vi "picoharp_initialize_correlation.vi"(8 "error in (no error)":errorcluster, 11 "hydraharp in":refnum<class "picoharp.lvclass">) -> (0 "error out":errorcluster, 3 "hydraharp out":refnum<class "picoharp.lvclass">)   [LabVIEW 2015, in "picoharp.lvclass"]
uses:
  picoharp.lvclass
  picoharp.lvclass/picoharp.ctl
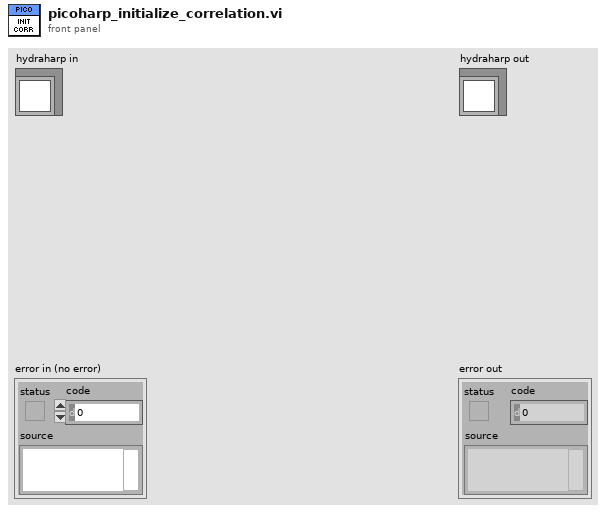
[diagram p1: front panel]
types:
  T1 = typedef "hydraharp_correlation_lag_settings.ctl" = cluster{"time_start":T2, "time_end":T2, "coarseness":i64}
  T2 = typedef "hydraharp_time_decades.ctl" = i64
  T3 = typedef "hydraharp_action_on_records.ctl" = enum16{"stream_to_file", "correlate", "stream to file and correlate", "histogram"}
  T4 = typedef "hpanel_acq_modes.ctl" = u16
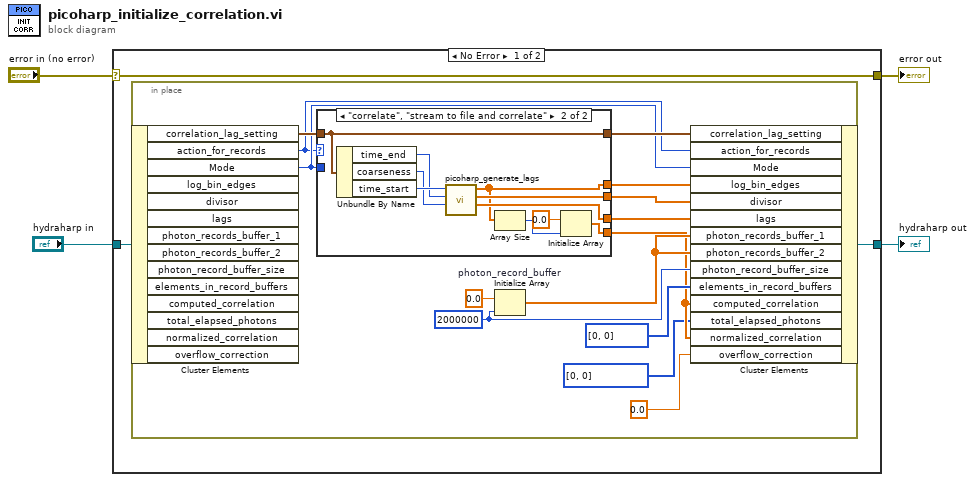
[diagram p0: block diagram]
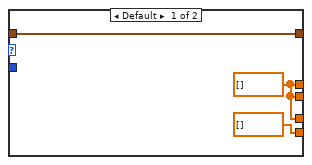
[diagram p2: hidden frame]
diagram:
  n1 = case shown="No Error" "error in (no error)" {
    selector: "error in (no error)" -> [w7 w36]
    tunnel: [w7 w36] -> w3
    tunnel: [w5 w35] -> w1
    tunnel: "hydraharp in" -> [w6 w35]
    frame No Error {
      n2 = in-place {
        w12 = 2000000 ("dimension size")
        n3 = in-place-cluster #1(w6) -> ("correlation_lag_setting"=w21:T1, "action_for_records"=w15:T3, "Mode"=w16:T4)  [unwired: 11 out]
        n4 = case shown="\"correlate\", \"stream to file and correlate\"" w15 {
          tunnel: w16 -> [_ _]
          tunnel: w21 -> [w24 w31]
          tunnel: [w24 w31] -> w20
          tunnel: [w23 w30] -> w19
          tunnel: [w23 w27] -> w18
          tunnel: [w23 w29] -> w17
          tunnel: [dbl[] [] w25] -> w10
          frame Default {
            w23 = dbl[] [] ("lags")
          }
          frame "correlate", "stream to file and correlate" {
            n5 = Unbundle By Name(w31) -> ("time_end"=w32:T2, "coarseness"=w33:i64, "time_start"=w34:T2)
            n6 = call "picoharp_generate_lags.vi"("coarseness"=w33, "time_end"=w32, "time_start"=w34) -> ("lags"=w29:dbl[], "divisor"=w30:dbl[], "log_bin_edges"=w27:dbl[])  [unwired: 6 in]
            n7 = Array Size(array=w27) -> (size(s)=w26:i32)
            n8 = Initialize Array(0.0 ("element"), w26) -> (w25:dbl[])
          }
        }
        n9 = Initialize Array "photon_record_buffer"(0.0 ("element"), w12) -> (w13:dbl[])
        n10 = in-place-cluster #1("correlation_lag_setting"=w20, "action_for_records"=w15, "Mode"=w16, "log_bin_edges"=w18, "divisor"=w19, "lags"=w17, "photon_records_buffer_1"=w13, "photon_records_buffer_2"=w13, "photon_record_buffer_size"=w12, "elements_in_record_buffers"=i32[] [0, 0], "computed_correlation"=w10, "total_elapsed_photons"=i32[] [0, 0], "normalized_correlation"=w10, "overflow_correction"=0.0) -> (w5:refnum<class "picoharp.lvclass">)
      }
    }
    frame Error {
    }
  }
  "error out" <- w3
  "hydraharp out" <- w1
